vi "Load Plugins from Disk.vi"(8 "error in (no error)":errorcluster, 11 "Plugin Location on Disk":path) -> (0 "error out":errorcluster, 3 "Array of Plugins":refnum<class "Generic Plugin.lvclass">[](array[class]))   [LabVIEW 2011, in "Plugin Load from Disk.lvclass"]
uses:
  Plugin Command Manager/Plugin Load from Disk/Plugin Load from Disk.lvclass
  Parent Plugin Definition/Plugin Template/Generic Plugin.lvclass
  Plugin Command Manager/Plugin Handler Launch Plugin/Plugin Handler Launch Plugin.lvclass
  Root Location Global.vi
  Plugin Command Manager/Plugin Handler Command.lvclass
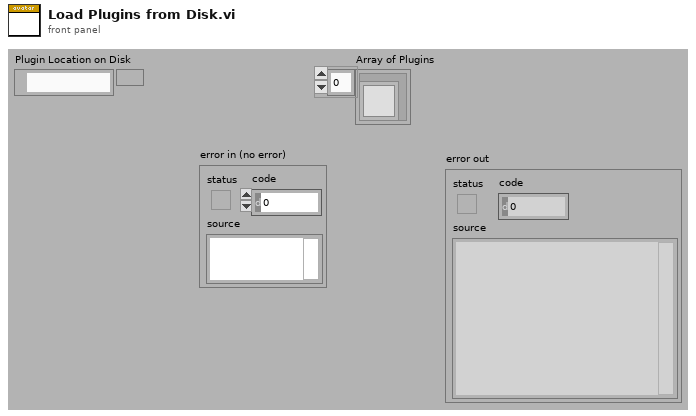
[diagram p1: front panel]
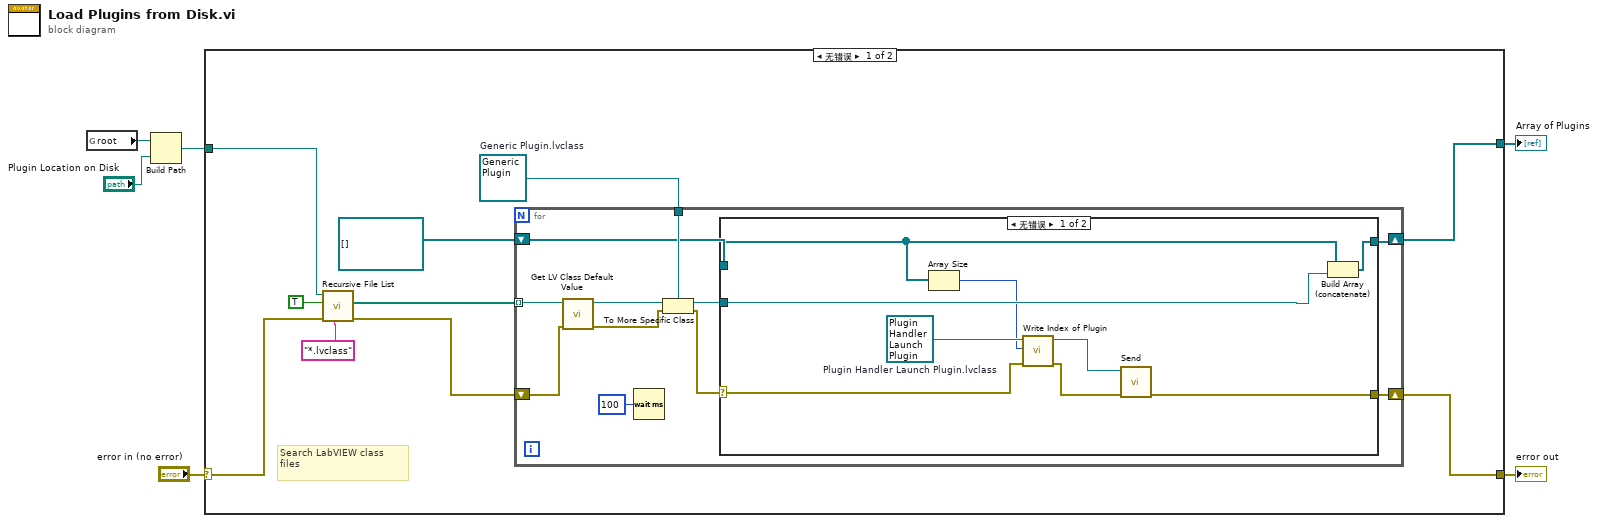
[diagram p0: block diagram]
diagram:
  n1 = global read "Root Location Global.vi" "root"() -> (w3:path)
  n2 = Build Path(base path=w3, name or relative path="Plugin Location on Disk") -> (appended path=w1:path)
  n3 = case shown="无错误" "error in (no error)" {
    selector: "error in (no error)" -> [w12 w39]
    tunnel: [w7 w39] -> w6
    tunnel: w1 -> [w13 _]
    tunnel: [w9 _] -> w4
    frame No Error {
      w11 = refnum<class "Generic Plugin.lvclass"> refnum  # Generic Plugin.lvclass
      # "Search LabVIEW class\nfiles"
      n4 = call <vilib>:"Recursive File List.vi"("pattern"="*.lvclass", "error in (no error)"=w12, "Treat LLBs as Folders?"=TRUE, "Folder Path"=w13) -> ("error out"=w8:errorcluster, "All Files in Dir"=w16:path[])  [unwired: 3 in, 3 out]
      n5 = for {
        tunnel: w16 -> [w27] mode=indexing
        tunnel: w11 -> [w25]
        shift-right: [w21] -> w9
        shift-left: refnum<class "Generic Plugin.lvclass">[] [] -> [w20]
        shift-right: [w18] -> w7
        shift-left: w8 -> [w19]
        n6 = call <vilib>:"Get LV Class Default Value.vi"("error in (no error)"=w19, "class path"=w27) -> ("error out"=w24:errorcluster, "object"=w26:refnum<class>)  [unwired: 8 in]
        n7 = Wait (ms)(milliseconds to wait=u32 100) -> ()  [unwired: 1 out]
        n8 = To More Specific Class(target class=w25, reference=w26, error in=w24) -> (specific class reference=w22:refnum<class "Generic Plugin.lvclass">, error out=w23:errorcluster)
        n9 = case shown="无错误" w23 {
          selector: w23 -> [w33 w37]
          tunnel: w22 -> [w34 _]
          tunnel: [w36 w38] -> w21
          tunnel: w20 -> [w32 w38]
          tunnel: [w35 w37] -> w18
          frame No Error {
            w31 = refnum<class "Plugin Handler Launch Plugin.lvclass"> refnum  # Plugin Handler Launch Plugin.lvclass
            n10 = Array Size(array=w32) -> (size(s)=w28:i32)
            n11 = call-dynamic "Write Index of Plugin.vi"("error in (no error)"=w33, "Index of Plugin"=w28, "Plugin Handler Launch Plugin in"=w31) -> ("error out"=w29:errorcluster, "Plugin Handler Launch Plugin out"=w30:refnum<class "Plugin Handler Launch Plugin.lvclass">)  [unwired: 7 in]
            n12 = call "Send.vi"("error in (no error)"=w29, "Plugin Generic Command in"=w30) -> ("error out"=w35:errorcluster)  [unwired: 8 in, 1 out]
            n13 = Build Array (concatenate)(w32, w34) -> (w36:refnum<class "Generic Plugin.lvclass">[])
          }
          frame Error {
          }
        }
      }
    }
    frame Error {
    }
  }
  "error out" <- w6
  "Array of Plugins" <- w4
